vi "Random Permutation.vi"(6 "seed":i32=-1, 7 "reset":bool, 10 "start":i32=1, 11 "N":u32=100) -> (0 "error":i32, 3 "random permutation":i32[](array[numeric]))   [LabVIEW 2017, in "NI_Gmath.lvlib"]
doc: "Generates random values from a variate X, where X describes the selected distribution type. You must manually select the polymorphic instance to use."
uses:
  NI_Gmath.lvlib
  Riffle Array (DBL).vi
  NI_AALBase.lvlib
panel:
  # "Random Permutation"
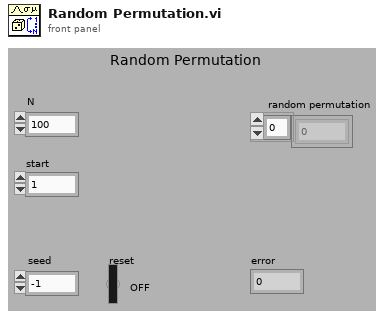
[diagram p1: front panel]
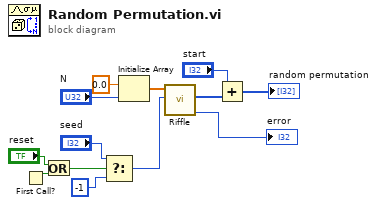
[diagram p0: block diagram]
diagram:
  n1 = First Call?() -> (First Call?: T/F=w13:bool)
  n2 = Or(x="reset", y=w13) -> (x .or. y?=w12:bool)
  n3 = Select(t="seed", s=w12, f=-1) -> (s? t:f=w8:i32)
  n4 = Initialize Array(0.0 ("element"), "N") -> (w2:dbl[])
  n5 = call-poly "Riffle.vi"("seed"=w8, "X"=w2) -> ("error"=→"error":i32, "Riffled Index"=w6:i32[])  [unwired: 7 in, 1 out]
  n6 = Add(x="start", y=w6) -> (x+y=→"random permutation":i32[])
